vi "WPI_UtilitiesRunCommand.vi"(9 "String Array":string[](array[string]), 11 "VI in":refnum<vi>) -> (3 "VI out":refnum<vi>)   [LabVIEW 2017]
panel:
  out "error out":errorcluster
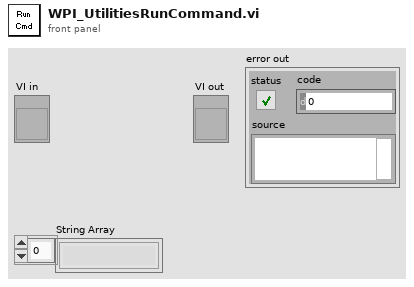
[diagram p1: front panel]
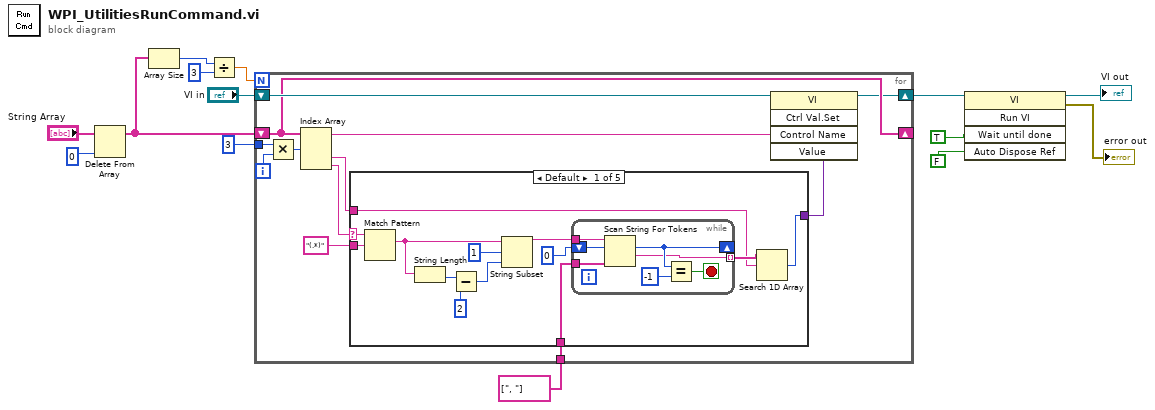
[diagram p0: block diagram]
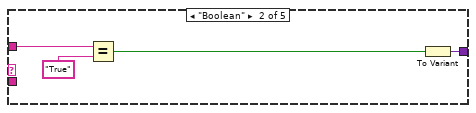
[diagram p2: hidden frame]
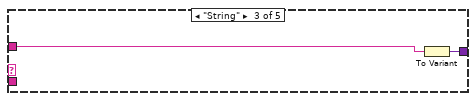
[diagram p3: hidden frame]
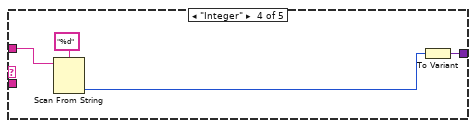
[diagram p4: hidden frame]
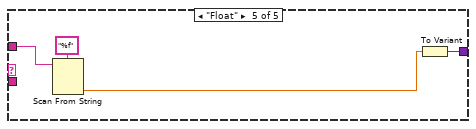
[diagram p5: hidden frame]
diagram:
  n1 = Delete From Array(array="String Array", index=0) -> (array with subset deleted=w8:string[])  [unwired: 1 in, 1 out]
  n2 = Array Size(array=w8) -> (size(s)=w10:i32)
  n3 = Divide(x=w10, y=3) -> (x/y=w13:dbl)
  n4 = for {
    N: w13 -> [_]
    shift-right: [w21] -> _
    shift-left: w8 -> [w21]
    tunnel: 3 -> [w22]
    shift-right: [w17] -> w4
    shift-left: "VI in" -> [w26]
    tunnel: string[] [", "] ("delimiters (\\s,\\t,\\r,\\n)") -> [w16]
    i -> [w23]
    n5 = Multiply(x=w22, y=w23) -> (x*y=w24:i32)
    n6 = Index Array(array=w21, index #1=w24) -> (element #1=w25:string, element #2=w19:string, element #3=w20:string)  [unwired: 2 in]
    n7 = case shown="Default" w20 {
      selector: w20 -> [w32 _ _ _ _]
      tunnel: w19 -> [w28 w50 w52 w56 w60]
      tunnel: [w27 w47 w51 w53 w58] -> w18
      tunnel: w16 -> [w39 _ _ _ _]
      tunnel: "(.*)" -> [w30 _ _ _ _]
      frame Default {
        n8 = Match Pattern(string=w32, regular expression=w30) -> (match substring=w34:string)  [unwired: 1 in, 3 out]
        n9 = String Length(string=w34) -> (length=w37:i32)
        n10 = Subtract(x=w37, y=2 ("offset (0)")) -> (x-y=w35:i32)
        n11 = String Subset(string=w34, offset (0)=1, length (rest)=w35) -> (substring=w31:string)
        n12 = while {
          tunnel: w31 -> [w46]
          shift-right: [w42] -> _
          shift-left: 0 ("offset past token") -> [w45]
          tunnel: w39 -> [w44]
          tunnel: [w40] -> w29 mode=indexing
          stop <- w43 stop-if-true
          n13 = Scan String For Tokens(6:w44, 8:w45, 9:w46) -> (1:w40:string, 2:w42:i32)  [unwired: 3 in, 2 out]
          n14 = Equal?(x=w42, y=-1) -> (x = y?=w43:bool)
        }
        n15 = Search 1D Array(1D array=w29, element=w28) -> (index of element=w27:i32)  [unwired: 1 in]
      }
      frame "Boolean" {
        n16 = Equal?(x=w50, y="True") -> (x = y?=w48:bool)
        n17 = To Variant(anything=w48) -> (Variant=w47:variant)
      }
      frame "String" {
        n18 = To Variant(anything=w52) -> (Variant=w51:variant)
      }
      frame "Integer" {
        n19 = Scan From String(format string="%d", input string=w56) -> (output 1=w54:i32)  [unwired: 3 in, 3 out]
        n20 = To Variant(anything=w54) -> (Variant=w53:variant)
      }
      frame "Float" {
        n21 = Scan From String(format string="%f", input string=w60) -> (output 1=w57:dbl)  [unwired: 3 in, 3 out]
        n22 = To Variant(anything=w57) -> (Variant=w58:variant)
      }
    }
    n23 = invoke class="VI" method="Ctrl Val.Set"(reference=w26, "Control Name"=w25, "Value"=w18) -> (reference out=w17:refnum<vi>)  [unwired: 2 in, 4 out]
  }
  n24 = invoke class="VI" method="Run VI"(reference=w4, "Wait until done"=TRUE ("Wait Until Done"), "Auto Dispose Ref"=FALSE ("Wait Until Done")) -> (reference out=→"VI out":refnum<vi>, error out=→"error out":errorcluster)  [unwired: 2 in, 3 out]
